vi "Wheel Info.vi"(8 "Wheel Diameter":dbl, 10 "Encoder Period":dbl, 11 "Encoder Position":dbl) -> (1 "Wheel Speed":dbl, 2 "Wheel Position":dbl)   [LabVIEW 2016]
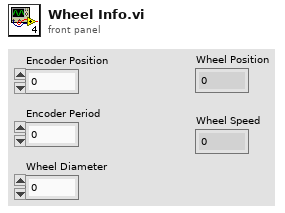
[diagram p1: front panel]
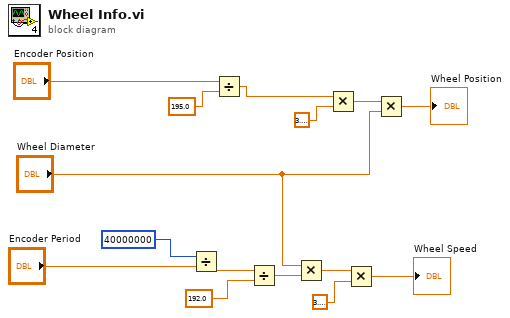
[diagram p0: block diagram]
diagram:
  n1 = Divide(x=40000000, y="Encoder Period") -> (x/y=w15:dbl)
  n2 = Divide(x="Encoder Position", y=195.0) -> (x/y=w3:dbl)
  n3 = Divide(x=w15, y=192.0) -> (x/y=w11:dbl)
  n4 = Multiply(x="Wheel Diameter", y=w11) -> (x*y=w10:dbl)
  n5 = Multiply(x=w3, y=3.141592653589793) -> (x*y=w5:dbl)
  n6 = Multiply(x=w10, y=3.141592653589793) -> (x*y=→"Wheel Speed":dbl)
  n7 = Multiply(x=w5, y="Wheel Diameter") -> (x*y=→"Wheel Position":dbl)
